vi "showHideVI.vi"(10 "VIname":string, 11 "showHide":bool) -> ()   [LabVIEW 2018]
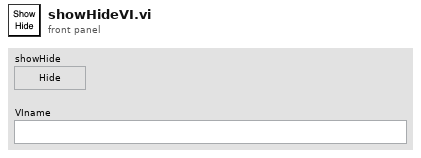
[diagram p1: front panel]
types:
  T1 = enum32{"Invalid", "Standard", "Closed", "Hidden", "Minimized", "Maximized"}
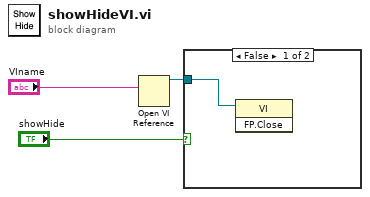
[diagram p0: block diagram]
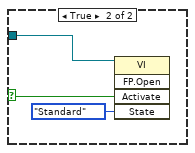
[diagram p2: hidden frame]
diagram:
  n1 = Open VI Reference(vi path="VIname") -> (vi reference=w2:refnum<vi>)  [unwired: 5 in, 1 out]
  n2 = case shown="False" "showHide" {
    selector: "showHide" -> [_ w5]
    tunnel: w2 -> [w4 w7]
    frame False {
      n3 = invoke class="VI" method="FP.Close"(reference=w4) -> ()  [unwired: 2 in, 3 out]
    }
    frame True {
      n4 = invoke class="VI" method="FP.Open"(reference=w7, "Activate"=w5, "State"=T1."Standard") -> ()  [unwired: 2 in, 5 out]
    }
  }
